vi "Pass If Equal Array.vi"(6 "delta (optional)":ext, 7 "custom report message (\"\")":string, 8 "error in (no error)":errorcluster, 9 "y":ext[](array[numeric]), 10 "x":ext[](array[numeric]), 11 "TestCase in":refnum<class "TestCase.lvclass">) -> (0 "error out":errorcluster, 3 "TestCase out":refnum<class "TestCase.lvclass">)   [LabVIEW 2015, in "VITAC.lvlib"]
uses:
  VITAC.lvlib
  <vilib>/addons/_JKI Toolkits/VI Tester/TestCase.llb/TestCase.lvclass
  <vilib>/addons/JSON API/Get Polymorphic/JSON GetSet.lvlib
  <vilib>/addons/JSON API/Variant JSON/Variant to JSON.vi
  <vilib>/addons/JSON API/Variant JSON/Variant JSON.lvlib
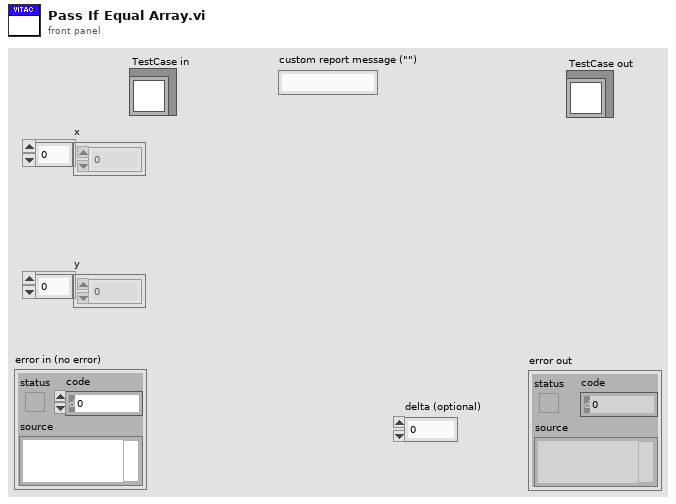
[diagram p1: front panel]
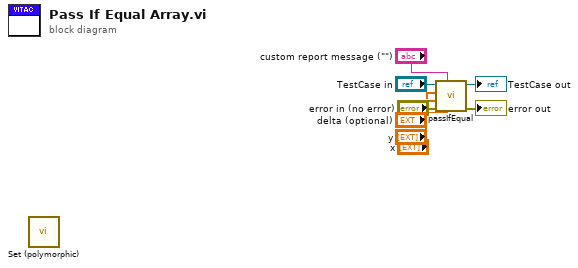
[diagram p0: block diagram]
diagram:
  n1 = call-poly <vilib>:"Set (polymorphic).vi"() -> ()  [unwired: 10 in, 2 out]
  n2 = call-dynamic "passIfEqual.vi"("delta (optional)"="delta (optional)", "custom report message (\"\")"="custom report message (\"\")", "error in (no error)"="error in (no error)", "y"="y", "x"="x", "TestCase in"="TestCase in") -> ("error out"=→"error out":errorcluster, "TestCase out"=→"TestCase out":refnum<class "TestCase.lvclass">)  [unwired: 4 in]
